vi "Create Evaluations.vi"(8 "error in (no error)":errorcluster, 11 "TDSCDMA_MODACC in":refnum<class "TDSCDMA_MODACC.lvclass">) -> (0 "error out":errorcluster, 2 "Evaluations Out":T1[](array[typedef]) {"Low Limit" format="%#_13g"; "SI Scaling" items=["femto"=-15, "pico"=-12, "nano"=-9, "micro"=-6, "milli"=-3, "percent"=-2, ""=0, "kilo"=3, "mega"=6, "giga"=9, "tera"=12]}, 3 "TDSCDMA_MODACC out":refnum<class "TDSCDMA_MODACC.lvclass">)   [LabVIEW 2016, in "SeqAuto Evaluations.lvlib" / "TDSCDMA_MODACC.lvclass"]
uses:
  TDSCDMA_MODACC.lvclass
  C:/projects/STS/Common/Sequence Automation/Plugins/SeqAuto IEvaluation.lvlibp/SeqAuto IEvaluation.lvclass
  Plugins/TestStand API Tools (TSAT).lvlibp/Evaluation Actions/Includes/Controls/TSAT Evaluation.ctl
  Plugins/TestStand API Tools (TSAT).lvlibp/Evaluation Actions/Includes/Controls/TSAT Eval SI Unit Scaling.ctl
  Plugins/TestStand API Tools (TSAT).lvlibp/Evaluation Actions/Includes/Controls/TSAT Evaluation Type.ctl
  Plugins/SeqAuto IEvaluation.lvlibp/Read Measurement Name.vi
  Plugins/TestStand API Tools (TSAT).lvlibp/Evaluation Actions/TSAT Evaluation Actions.lvlib
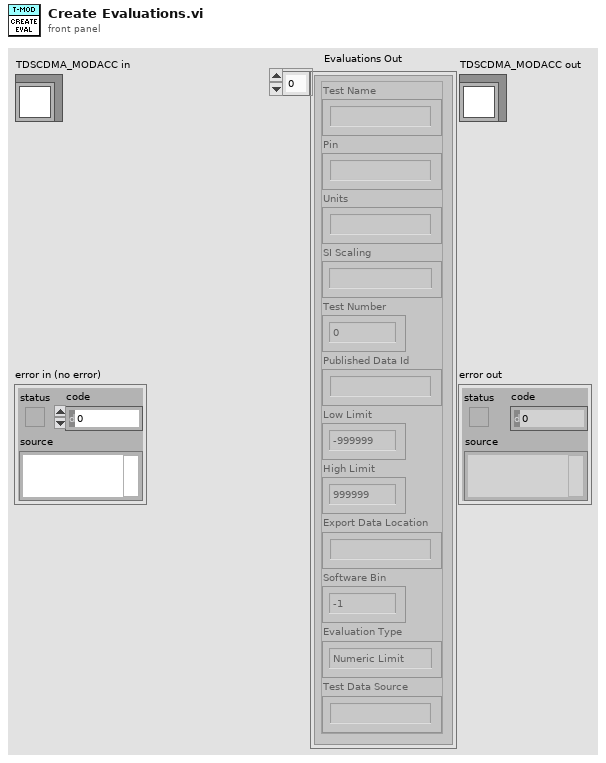
[diagram p1: front panel]
types:
  T1 = typedef "TestStand API Tools (TSAT).lvlibp/TSAT Evaluation Actions.lvlib/TSAT Evaluation.ctl" = cluster{"Test Name":string, "Pin":string, "Units":string, "SI Scaling":T2, "Test Number":i32, "Published Data Id":string, "Low Limit":dbl, "High Limit":dbl, "Export Data Location":string, "Software Bin":i64, "Evaluation Type":T3, "Test Data Source":string}
  T2 = typedef "TestStand API Tools (TSAT).lvlibp/TSAT Evaluation Actions.lvlib/TSAT Eval SI Unit Scaling.ctl" = i16
  T3 = typedef "TestStand API Tools (TSAT).lvlibp/TSAT Evaluation Actions.lvlib/TSAT Evaluation Type.ctl" = enum16{"Numeric Limit", "Pass/Fail", "None"}
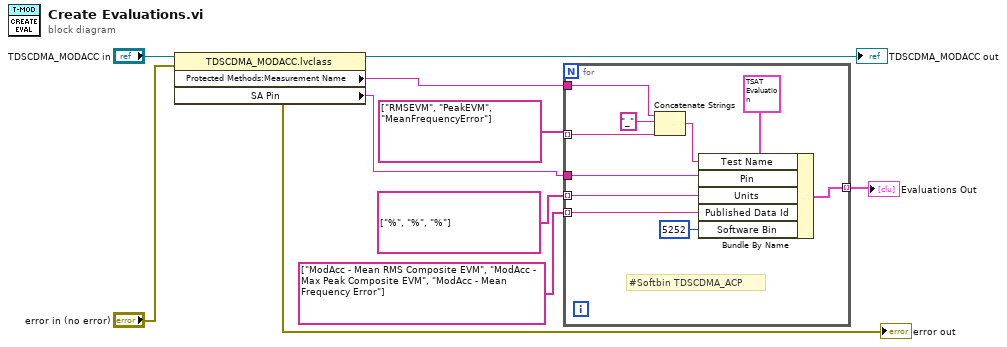
[diagram p0: block diagram]
diagram:
  n1 = property class="TDSCDMA_MODACC.lvclass"(reference="TDSCDMA_MODACC in", error in="error in (no error)") -> (reference out=→"TDSCDMA_MODACC out":refnum<class "TDSCDMA_MODACC.lvclass">, error out=→"error out":errorcluster, "Protected Methods:Measurement Name"=w3:string, "SA Pin"=w2:string)
  n2 = for {
    tunnel: string[] ["%", "%", "%"] -> [w19] mode=indexing
    tunnel: string[] ["RMSEVM", "PeakEVM", "MeanFrequencyError"] -> [w18] mode=indexing
    tunnel: string[] ["ModAcc - Mean RMS Composite EVM", "ModAcc - Max Peak Composite EVM", "ModAcc - Mean Frequency Error"] ("Array") -> [w15] mode=indexing
    tunnel: [w14] -> w1 mode=indexing
    tunnel: w3 -> [w13]
    tunnel: w2 -> [w12]
    # "#Softbin TDSCDMA_ACP"
    n3 = Concatenate Strings(w13, "_" ("string"), w18) -> (w17:string)
    n4 = Bundle By Name(cluster=T1 {"Test Name"="", "Pin"="", "Units"="", "SI Scaling"=0, "Test Number"=0, "Published Data Id"="", "Low Limit"=-999999.0, "High Limit"=999999.0, "Export Data Location"="", "Software Bin"=-1, "Evaluation Type"=enum."Numeric Limit", "Test Data Source"=""} ("Evaluation"), "Test Name"=w17, "Pin"=w12, "Units"=w19, "Published Data Id"=w15, "Software Bin"=i64 5252) -> (w14:T1)
  }
  "Evaluations Out" <- w1
